vi "Retrieve Calibration Data.vi"(0 "Calibration Signal Path Name":string="sg_to_dut", 11 "error in (no error)":errorcluster, 12 "Folder Path":path) -> (6 "Calibration Data":T1 {"Calibration Table" min=0.0 max=127.0 format="%.2p"; "Time Stamp, sec" format="%^.2e"; "Temperature, C" format="%.1f"}, 15 "error out":errorcluster)   [LabVIEW 2011]
doc: "This utility retrieves the calibration data from an .tdms file. \nString name get converted to a file path relative to the VIs path.\n\n(c) Copyright 2006, National Instruments, Inc. This VI may not be duplicated, sold, or distributed without written consent from National Instruments."
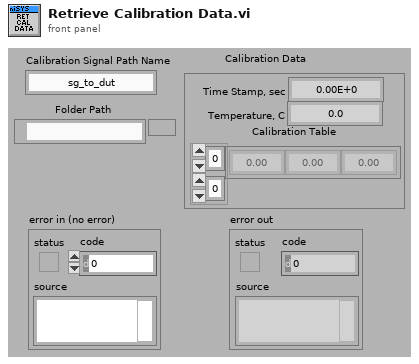
[diagram p1: front panel]
types:
  T1 = cluster{"Temperature, C":dbl, "Time Stamp, sec":dbl, "Calibration Table":dbl[][]}
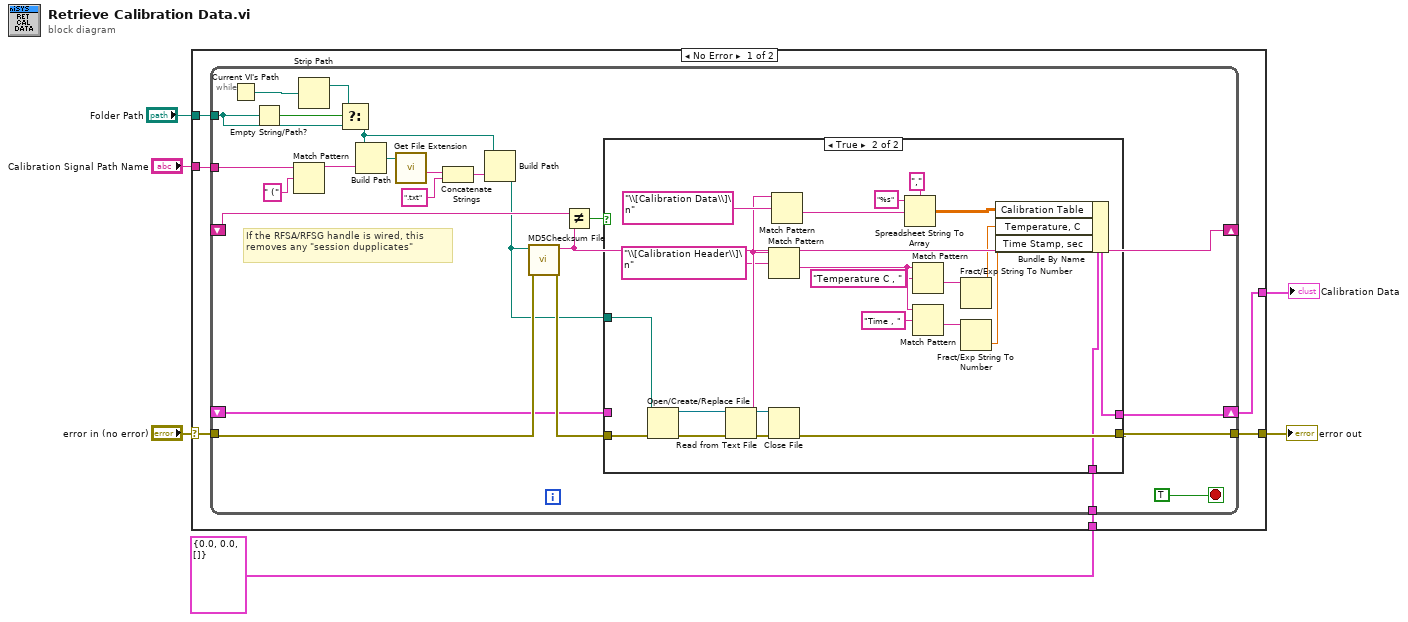
[diagram p0: block diagram]
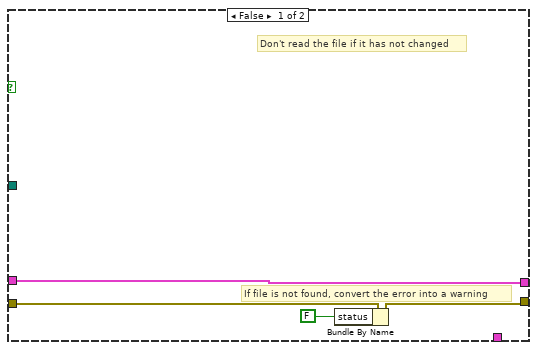
[diagram p2: hidden frame]
diagram:
  n1 = case shown="No Error" "error in (no error)" {
    selector: "error in (no error)" -> [w12 w63]
    tunnel: [w11 w63] -> w5
    tunnel: "Calibration Signal Path Name" -> [w9 _]
    tunnel: [w10 _] -> w1
    tunnel: T1 {"Temperature, C"=0.0, "Time Stamp, sec"=0.0, "Calibration Table"=[]} ("Calibration Data") -> [w8 _]
    tunnel: "Folder Path" -> [w7 _]
    frame No Error {
      n2 = while {
        tunnel: w12 -> [w32]
        tunnel: [w21] -> w11
        shift-right: [w33] -> _
        shift-left: _ -> [w34]
        tunnel: w9 -> [w14]
        shift-right: [w22] -> w10
        shift-left: _ -> [w24]
        tunnel: w8 -> [w23]
        tunnel: w7 -> [w19]
        stop <- TRUE stop-if-true
        # "If the RFSA/RFSG handle is wired, this removes any \"session dupplicates\""
        n3 = Current VI's Path() -> (path=w17:path)
        n4 = Empty String/Path?(string/path=w19) -> (empty?=w20:bool)
        n5 = Match Pattern(string=w14, regular expression=" (") -> (before substring=w13:string)  [unwired: 1 in, 3 out]
        n6 = Strip Path(path=w17) -> (stripped path=w16:path)  [unwired: 1 out]
        n7 = Select(t=w16, s=w20, f=w19) -> (s? t:f=w18:path)
        n8 = Build Path(base path=w18, name or relative path=w13) -> (appended path=w31:path)
        n9 = call <vilib>:"Get File Extension.vi"("file"=w31) -> ("filename without extension"=w30:string)  [unwired: 1 in, 9 out]
        n10 = Concatenate Strings(w30, ".txt" ("string")) -> (w28:string)
        n11 = Build Path(base path=w18, name or relative path=w28) -> (appended path=w25:path)
        n12 = call <vilib>:"MD5Checksum File.vi"("error in (no error)"=w32, "Path"=w25) -> ("error out"=w26:errorcluster, "MD5 message-digest"=w33:string)  [unwired: 8 out]
        n13 = Not Equal?(x=w34, y=w33) -> (x != y?=w27:bool)
        n14 = case shown="True" w27 {
          tunnel: [w37 w42] -> w21
          tunnel: w25 -> [_ w44]
          tunnel: w26 -> [w38 w43]
          tunnel: [w36 w41] -> w22
          tunnel: w23 -> [_ w40]
          tunnel: w24 -> [w36 _]
          frame False {
            # "If file is not found, convert the error into a warning"
            # "Don't read the file if it has not changed"
            n15 = Bundle By Name(cluster=w38, "status"=FALSE) -> (w37:errorcluster)
          }
          frame True {
            n16 = Open/Create/Replace File(file path (use dialog)=w44, error in=w43) -> (refnum out=w45:refnum<file>, error out=w46:errorcluster)  [unwired: 4 in, 1 out]
            n17 = Read from Text File(file (use dialog)=w45, error in=w46) -> (refnum out=w47:refnum<file>, text=w50:string, error out=w48:errorcluster)  [unwired: 2 in, 1 out]
            n18 = Match Pattern(string=w50, regular expression="\\[Calibration Header\\]\n") -> (after substring=w60:string)  [unwired: 1 in, 3 out]
            n19 = Close File(refnum=w47, error in=w48) -> (error out=w42:errorcluster)  [unwired: 1 out]
            n20 = Match Pattern(string=w50, regular expression="\\[Calibration Data\\]\n") -> (after substring=w52:string)  [unwired: 1 in, 3 out]
            n21 = Spreadsheet String To Array(delimiter (Tab)=",", format string="%s", spreadsheet string=w52) -> (array=w55:dbl[][])  [unwired: 1 in]
            n22 = Match Pattern(string=w60, regular expression="Temperature C , ") -> (after substring=w57:string)  [unwired: 1 in, 3 out]
            n23 = Match Pattern(string=w60, regular expression="Time , ") -> (after substring=w59:string)  [unwired: 1 in, 3 out]
            n24 = Fract/Exp String To Number(string=w57) -> (number=w58:dbl)  [unwired: 3 in, 1 out]
            n25 = Fract/Exp String To Number(string=w59) -> (number=w62:dbl)  [unwired: 3 in, 1 out]
            n26 = Bundle By Name(cluster=w40, "Calibration Table"=w55, "Temperature, C"=w58, "Time Stamp, sec"=w62) -> (w41:T1)
          }
        }
      }
    }
    frame Error {
    }
  }
  "error out" <- w5
  "Calibration Data" <- w1
